vi "RT Main.vi"() -> ()   [LabVIEW 2011]
doc: "This example shows how to use Simulation Module and Control Design Toolkit together and how to transfer the controller from Design to Simulation. It also uses the 3D Picture Control Toolkit to animate the system.\nThis example is derived from the Quanser (www.quanser.com) 3 DOF Helicopter academic experiment."
uses:
  RT States.ctl
  <vilib>/Simulation/Scripting/Companion Diagram/SimConfigNode/SimParams.ctl
  <vilib>/Simulation/Scripting/Companion Diagram/SimConfigNode/_simSolvers.ctl
  <vilib>/Simulation/Implementation/Shared/SIMSCR Execution Mode.ctl
  <vilib>/Platform/TimedLoop/XDataNode/timing_clust.ctl
  <vilib>/Platform/TimedLoop/XDataNode/nitl_modes.ctl
  <vilib>/Platform/TimedLoop/XDataNode/wakeup.ctl
  <vilib>/Simulation/Param Hierarchy/Typedefs/SIMPH Param Control Actions.ctl
  <vilib>/Simulation/Scripting/Editor Utilities/SIM subVI tag data.ctl
  <vilib>/Simulation/Scripting/Editor Utilities/SIM subVI execution type.ctl
  <vilib>/Simulation/Implementation/Shared/NILVSim_FinishedLate.vi
  <vilib>/Simulation/Utility/Implementation/SIM Halt.vi
  <vilib>/Simulation/SignalArithmetic/Implementation/NILVSim Gain.llb/SIM Gain (scalar).vi
  <vilib>/Simulation/Implementation/Shared/SIM Fire Discrete SubVI.vi
  <vilib>/Simulation/Implementation/Shared/NILVSim_Manager.vi
  <vilib>/Simulation/Implementation/Shared/NILVSim_ParamChanged.vi
  <vilib>/Simulation/Implementation/Shared/NILVSim_FinalizeModel.vi
  <vilib>/Simulation/Implementation/Shared/SIM Fire Discrete SubVI (Core).vi
  MyGlobal.vi
  <vilib>/FPGAPlugInAG/sbRIO-9642/niLvFpga_Open_sbRIO-9642.vi
  <vilib>/Utility/error.llb/Error Cluster From Error Code.vi
  <vilib>/rvi/errors/niLvFpgaAdjustHostInterfaceError.vi
  <vilib>/FPGAPlugInAG/sbRIO-9642/niLvFpga_Reset_sbRIO-9642.vi
  <vilib>/FPGAPlugInAG/sbRIO-9642/niLvFpga_Run_sbRIO-9642.vi
  <vilib>/Simulation/Implementation/Shared/SIM Unbundle Sim Info.vi
  <vilib>/Simulation/Implementation/Shared/NILVSim_GetModelError.vi
  <vilib>/Simulation/Implementation/Shared/SIM Bundle Sim Info.vi
  <vilib>/Simulation/Implementation/Shared/NILVSim_Initialize.vi
  PWM to Set.vi
  Set to PWM.vi
  <vilib>/FPGAPlugInAG/sbRIO-9642/niLvFpga_Close_sbRIO-9642.vi
  <vilib>/rvi/interface/nirviOpenFPGA/nirviOpenFPGA.xnode
  FPGA Bitfiles/sbRIOController.lv~4B_sbRIO-9642_FPGA Main NoStartE~C3.lvbitx
  <vilib>/rvi/interface/nirviReadWriteControl/nirviReadWriteControl.xnode
  <vilib>/rvi/interface/nirviMethod/nirviMethod.xnode
  <vilib>/Simulation/Scripting/Companion Diagram/SimConfigNode/SimDog.xnode
  Heli SubVIs/cdex_Elevation PID.vi
  Heli SubVIs/cdex_Pitch PID.vi
  Heli SubVIs/cdex_Position PID.vi
  <vilib>/Platform/TimedLoop/XDataNode/XDataNode.xnode
  <vilib>/Simulation/Implementation/XNodeFramework/SimXNode/SimX.xnode
  <vilib>/rvi/interface/nirviCloseFPGA/nirviCloseFPGA.xnode
  NiFpgaLv.dll
  <vilib>/Platform/TimedLoop/XDataNode/XDNodeRunTimeDep.lvlib
  <vilib>/Simulation/Implementation/Shared/NI_SIM_Implementation.lvlib
panel:
  out "error out":errorcluster
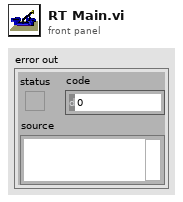
[diagram p1: front panel]
types:
  T1 = typedef "RT States.ctl" = enum16{"Passive", "Active"}
  T2 = typedef "SIMPH Param Control Actions.ctl" = enum16{"get params", "set params"}
  T3 = typedef "SIM subVI tag data.ctl" = cluster{"period":dbl, "skew":dbl, "Simulation execution type":T4}
  T4 = typedef "SIM subVI execution type.ctl" = enum16{"Function call", "Discrete", "Continuous", "Initialization only", "Final step only"}
  T5 = typedef "XDNodeRunTimeDep.lvlib/timing_clust.ctl" = cluster{"Expected End [f-1]":u64, "Actual End [f-1]":u64, "Finished Late? [f-1]":bool, "Expected End [i-1]":u64, "Actual End [i-1]":u64, "Finished Late? [i-1]":bool, "Expected Start [i]":u64, "Actual Start [i]":u64, "Expected Start [f]":u64, "Actual Start [f]":u64, "Source Name":string, "Structure Name":string, "Period":i64, "Deadline":i64, "Offset":i64, "Start":i64, "Priority":i32, "Timeout":i32, "Mode":T6, "Wakeup Reason":T7, "Error":errorcluster, "Source Type":string, "Secondary Source Type":string, "Global End Time":u64, "Global Start Time":u64, "Frame Duration":u64, "Iteration Duration":u64, "Assigned CPU":i32, "I/O Scan Engine Mode":u32}
  T6 = typedef "XDNodeRunTimeDep.lvlib/nitl_modes.ctl" = enum32{"No Change", "Process missed periods, maintain original phase", "Discard missed periods, maintain original phase", "Process missed periods, ignore original phase", "Discard missed periods, ignore original phase"}
  T7 = typedef "XDNodeRunTimeDep.lvlib/wakeup.ctl" = enum32{"Normal", "Aborted", "Asynchronous wakeup", "Timing source error", "Timed loop error", "Timeout"}
  T8 = typedef "SimParams.ctl" = cluster{"Initial Time (s)":dbl, "Final Time (s)":dbl, "Step Size (s)":dbl, "ODE Solver":T9, "Minimum Step Size (s)":dbl, "Maximum Step Size (s)":dbl, "Relative Tolerance":dbl, "Absolute Tolerance":dbl, "Software Timing":bool, "Initial Step Size (s)":dbl, "Automatic Fixed Step Size?":bool, "Automatic Discrete Step Size?":bool, "Discrete Step Size (s)":dbl, "Calculate using Time Step":bool, "Solver Wired?":bool, "Prev.Frm.Expected End":u64, "Prev.Frm.Actual End":u64, "Prev.Frm.Finished Late?":bool, "Prev.Iter.Expected End":u64, "Prev.Iter.Actual End":u64, "Prev.Iter.Finished Late?":bool, "Expected Iteration Start":u64, "Actual Iteration Start":u64, "Expected Frame Start":u64, "Actual Frame Start":u64, "Source Name":string, "Name":string, "Period":i64, "Deadline":i64, "Offset":i64, "Start":i64, "Priority":i32, "Timeout":i32, "Processor":i32, "Mode":enum32{"No Change", "Process missed periods, maintain original phase", "Discard missed periods, maintain original phase", "Process missed periods, ignore original phase", "Discard missed periods, ignore original phase"}, "Wakeup reason":enum32{"Normal", "Aborted", "Asynchronous wakeup", "Timing source error", "Timed loop error", "Timeout"}, "Error":errorcluster, "Source Type":string, "Secondary Source Type":string, "Global End Time":u64, "Global Start Time":u64, "Full Solver Reset":bool, "Execution Mode":T10, "Nan/Inf Check":bool, "Custom Solver Library":string, "Solver Is Variable":bool, "custom solver name":string}
  T9 = typedef "_simSolvers.ctl" = enum16{"Runge-Kutta 1 (Euler)", "Runge-Kutta 2", "Runge-Kutta 3", "Runge-Kutta 4", "Runge-Kutta 23 (variable)", "Runge-Kutta 45 (variable)", "BDF (variable)", "Adams-Moulton (variable)", "Rosenbrock (variable)", "Discrete States Only", "Linearizer", "State Query", "Trim Eval", "Custom Solver"}
  T10 = typedef "SIMSCR Execution Mode.ctl" = u16
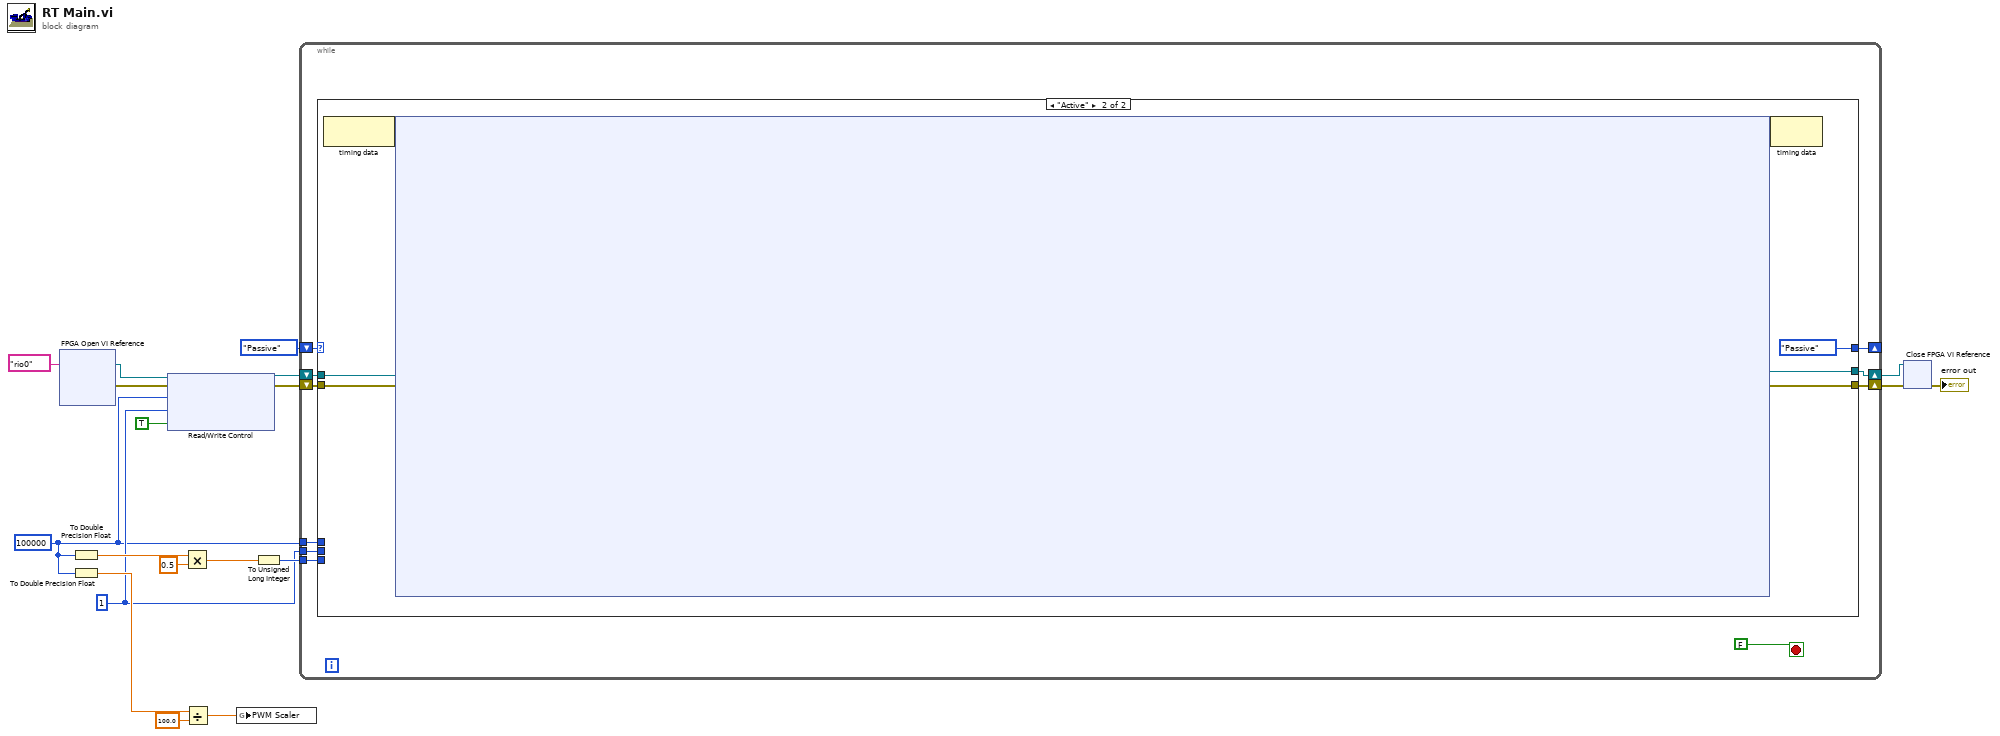
[diagram p0: block diagram]
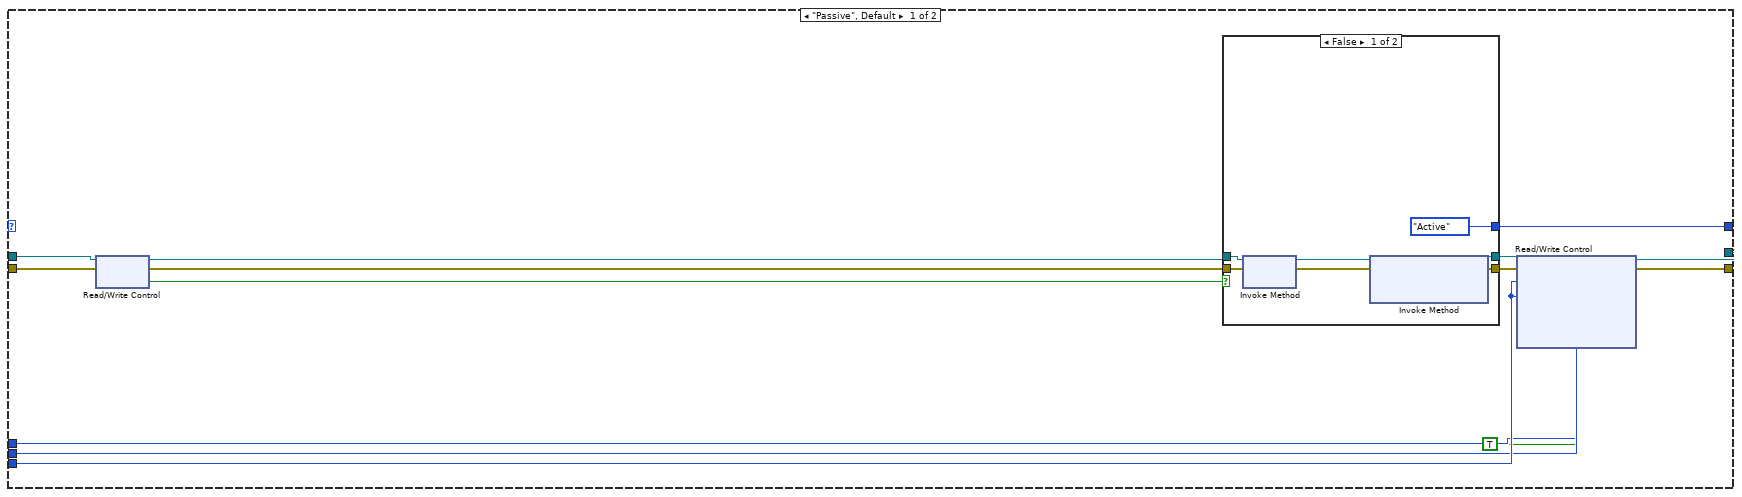
[diagram p2: hidden frame]
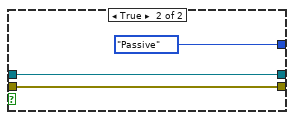
[diagram p3: hidden frame]
diagram:
  w4 = u16 1 ("Clock Divider (ticks)")
  w3 = u32 100000 ("PWM Period (ticks)")
  n1 = xnode "FPGA Open VI Reference"("resource name"=tag "rio0") -> ("FPGA VI Reference Out"=w18:refnum<k20>, "error out"=w19:errorcluster)  [unwired: 1 in]
  n2 = To Double Precision Float(number=w3) -> (double precision float=w10:dbl)
  n3 = To Double Precision Float(number=w3) -> (double precision float=w13:dbl)
  n4 = xnode "Read/Write Control"("FPGA VI Reference In"=w18, "error in"=w19, "PWM Period (ticks)"=w3, "Clock Divider"=w4, "ENC In Clock"=TRUE) -> ("FPGA VI Reference Out"=w2:refnum<k20>, "error out"=w7:errorcluster)
  n5 = Multiply(x=w10, y=0.5) -> (x*y=w11:dbl)
  n6 = Divide(x=w13, y=100.0) -> (x/y=w9:dbl)
  n7 = global write "MyGlobal.vi" "PWM Scaler"(w9) -> ()
  n8 = To Unsigned Long Integer(number=w11) -> (unsigned 32bit integer=w8:u32)
  n9 = while {
    shift-right: [w25] -> _
    shift-left: RT_States."Passive" ("Enum") -> [w23]
    tunnel: w8 -> [w27]
    shift-right: [w24] -> w6
    shift-left: w7 -> [w29]
    shift-right: [w20] -> w5
    shift-left: w2 -> [w28]
    tunnel: w4 -> [w22]
    tunnel: w3 -> [w21]
    stop <- FALSE ("stop") stop-if-true
    n10 = case shown="\"Active\"" w23 {
      tunnel: w29 -> [w43 w58]
      tunnel: w28 -> [w42 w57]
      tunnel: w27 -> [w33 _]
      tunnel: [w38 RT_States."Passive" ("Enum")] -> w25
      tunnel: [w34 w54] -> w24
      tunnel: [w35 w55] -> w20
      tunnel: w22 -> [w32 _]
      tunnel: w21 -> [w31 _]
      frame "Passive", Default {
        n11 = xnode "Read/Write Control"("FPGA VI Reference In"=w42, "error in"=w43) -> ("FPGA VI Reference Out"=w41:refnum<k20>, "error out"=w40:errorcluster, "Reset?"=w39:bool)
        n12 = case shown="False" w39 {
          tunnel: w41 -> [w50 w52]
          tunnel: w40 -> [w48 w53]
          tunnel: [w46 w53] -> w36
          tunnel: [w45 w52] -> w37
          tunnel: [RT_States."Active" ("Enum") RT_States."Passive" ("Enum")] -> w38
          frame False {
            n13 = xnode "Invoke Method"("FPGA VI Reference In"=w50, "error in"=w48) -> ("FPGA VI Reference Out"=w49:refnum<k20>, "error out"=w47:errorcluster)
            n14 = xnode "Invoke Method"("FPGA VI Reference In"=w49, "error in"=w47) -> ("FPGA VI Reference Out"=w45:refnum<k20>, "error out"=w46:errorcluster)  [unwired: 1 in]
          }
          frame True {
          }
        }
        n15 = xnode "Read/Write Control"("FPGA VI Reference In"=w37, "error in"=w36, "Fan High Time 1"=w33, "Fan High Time 2"=w33, "ENC In Clock"=TRUE, "PWM Period (ticks)"=w31, "Clock Divider"=w32) -> ("FPGA VI Reference Out"=w35:refnum<k20>, "error out"=w34:errorcluster)
      }
      frame "Active" {
        n16 = node-c288() -> (w60:variant)  [unwired: 1 in]
        n17 = node-c254 ("Simulation Loop")(w60, w58, w57) -> (w59:variant, w54:errorcluster, w55:refnum<k20>)
        n18 = node-c288(w59) -> ()  [unwired: 1 out]
      }
    }
  }
  n19 = xnode "Close FPGA VI Reference"("FPGA VI Reference In"=w5, "error in"=w6) -> ("error out"=→"error out":errorcluster)
